vi "subXMLGetSourceItemName.vi"(9 "index (1)":u32=1, 11 "Refnum in":refnum<k20>) -> (1 "Ref type?":bool, 3 "source name":string)   [LabVIEW 2019, in "SolutionBuilder.lvlib" / "SolutionBuilder.lvclass"]
uses:
  SolutionBuilder.lvclass
  <vilib>/xml/NI_XML.lvlib
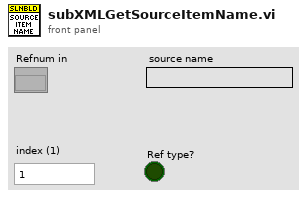
[diagram p1: front panel]
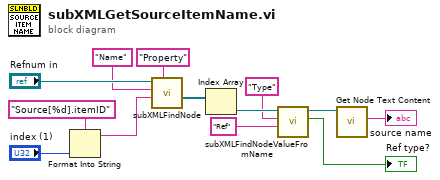
[diagram p0: block diagram]
diagram:
  n1 = Format Into String(format string="Source[%d].itemID" ("Property value"), "index (1)") -> (resulting string=w6:string)  [unwired: 2 in, 1 out]
  n2 = call "subXMLFindNode.vi"("Node name"="Property", "Property value"=w6, "Property name"="Name", "Refnum in"="Refnum in") -> ("Nodes"=w12:refnum<k20>[])  [unwired: 6 in, 1 out]
  n3 = Index Array(array=w12) -> (element=w4:refnum<k20>)  [unwired: 1 in]
  n4 = call "subXMLFindNodeValueFromName.vi"("Property value"="Ref" ("Property name"), "Property name"="Type", "Refnum in"=w4) -> ("Found?"=→"Ref type?":bool, "Refnum out"=w5:refnum<k20>)  [unwired: 6 in, 1 out]
  n5 = call <vilib>:"Get Node Text Content.vi"("node in"=w5) -> ("node text"=→"source name":string)  [unwired: 8 in, 2 out]
